vi "prep_PDS_plot.vi"(7 "RT PDS Data":cluster{dbl[], i32[], dbl[]}) -> (8 "RT PDS Data Sets":T1)   [LabVIEW 2023]
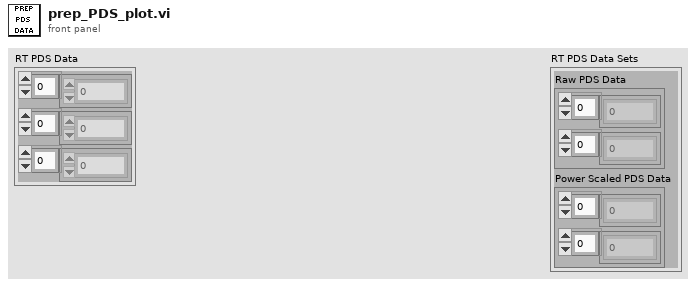
[diagram p1: front panel]
types:
  T1 = cluster{"Raw PDS Data":cluster{dbl[], dbl[]}, "Power Scaled PDS Data":cluster{dbl[], dbl[]}}
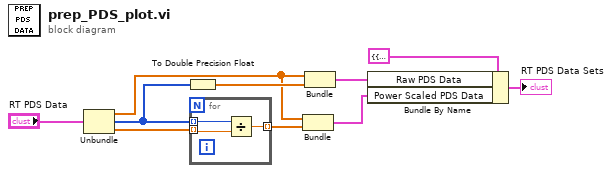
[diagram p0: block diagram]
diagram:
  n1 = Unbundle("RT PDS Data") -> (w6:dbl[], w8:i32[], w9:dbl[])
  n2 = To Double Precision Float(number=w8) -> (double precision float=w7:dbl[])
  n3 = for {
    tunnel: w8 -> [w13] mode=indexing
    tunnel: w9 -> [w12] mode=indexing
    tunnel: [w11] -> w5 mode=indexing
    n4 = Divide(x=w13, y=w12) -> (x/y=w11:dbl)
  }
  n5 = Bundle(w6, w5) -> (w2:cluster{dbl[], dbl[]})  [unwired: 1 in]
  n6 = Bundle(w6, w7) -> (w3:cluster{dbl[], dbl[]})  [unwired: 1 in]
  n7 = Bundle By Name(cluster=T1 {"Raw PDS Data"={[], []}, "Power Scaled PDS Data"={[], []}}, "Raw PDS Data"=w3, "Power Scaled PDS Data"=w2) -> (→"RT PDS Data Sets":T1)
